vi "User Status Updated.vi"(8 "error in (no error)":errorcluster, 10 "New User Status":string, 11 "UI Status Update in":refnum<class "Controller Update.lvclass">) -> (0 "error out":errorcluster, 3 "UI Status Update out":refnum<class "Controller Update.lvclass">)   [LabVIEW 2020, in "Interface.lvlib" / "Controller Update.lvclass"]
uses:
  Controller Update.lvclass
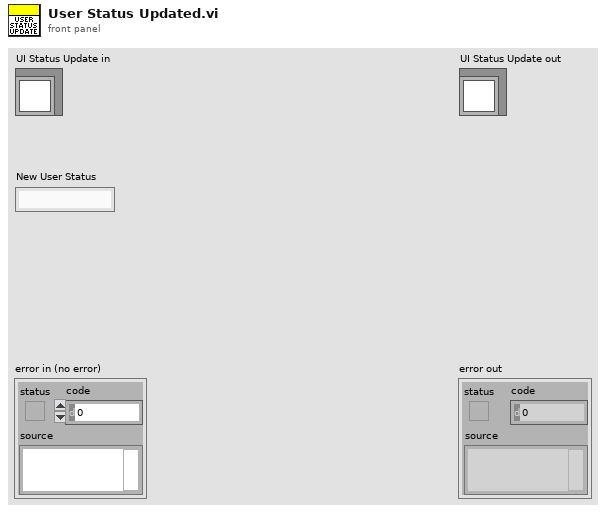
[diagram p1: front panel]
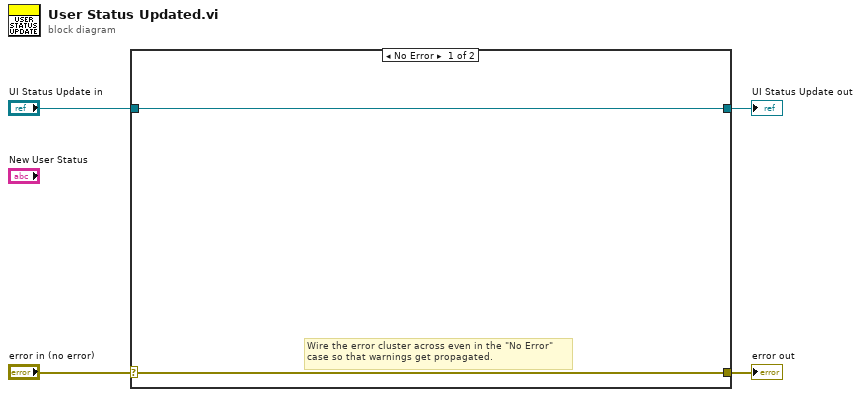
[diagram p0: block diagram]
diagram:
  n1 = case shown="No Error" "error in (no error)" {
    selector: "error in (no error)" -> [w5 w8]
    tunnel: [w5 w8] -> w3
    tunnel: [w6 w7] -> w1
    tunnel: "UI Status Update in" -> [w6 w7]
    frame No Error {
      # "Wire the error cluster across even in the \"No Error\"\ncase so that warnings get propagated."
    }
    frame Error {
    }
  }
  "error out" <- w3
  "UI Status Update out" <- w1
